vi "Get Template LVClasses.vi"(11 "LVLib":refnum<vi>) -> (2 "Class Ref Map":variant, 3 "LVLib Dup":refnum<vi>)   [LabVIEW 2013]
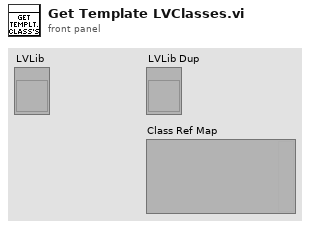
[diagram p1: front panel]
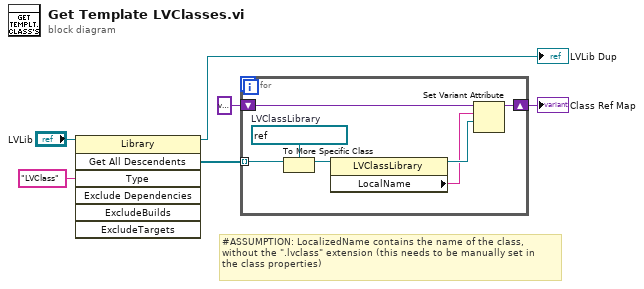
[diagram p0: block diagram]
diagram:
  # "#ASSUMPTION: LocalizedName contains the name of the class,\nwithout the \".lvclass\" extension (this needs to be manually set in\nthe class properties)"
  n1 = invoke class="Library" method="Get All Descendents"(reference="LVLib", "Type"="LVClass") -> (reference out=→"LVLib Dup":refnum<vi>, "All Descendents"=w3:refnum<vi>[])  [unwired: 5 in, 5 out]
  n2 = for {
    tunnel: w3 -> [w11] mode=indexing
    shift-right: [w8] -> w1
    shift-left: variant ("Class Ref Map") -> [w9]
    w13 = refnum<vi> refnum  # LVClassLibrary
    n3 = To More Specific Class(target class=w13, reference=w11) -> (specific class reference=w12:refnum<vi>)  [unwired: 1 in, 1 out]
    n4 = property class="LVClassLibrary"(reference=w12) -> (reference out=w10:refnum<vi>, "LocalName"=w7:string)  [unwired: 1 in, 1 out]
    n5 = Set Variant Attribute(Variant=w9, name=w7, value=w10) -> (Variant out=w8:variant)  [unwired: 1 in, 2 out]
  }
  "Class Ref Map" <- w1
